vi "Kikusui PLZ-Configure Operation Value.vi"(8 "error in":errorcluster, 9 "Values (0)":dbl format="%#.3g", 10 "Value Type (0:Current)":u16(ring) items=["Current", "Voltage", "Power", "Conductance"], 11 "Kikusui PLZ Setting In":T1={"VISA Resource Name"="", "Baud Rate"=19200, "Stop Bits"=20, "Wait For Read(ms)"=0} {"Stop Bits" items=["1.0"=10, "2.0"=20]; "Baud Rate" items=["2400"=2400, "4800"=4800, "9600"=9600, "19200"=19200]}) -> (0 "error out":errorcluster, 3 "Kikusui PLZ Setting Out":T1={"VISA Resource Name"="", "Baud Rate"=19200, "Stop Bits"=20, "Wait For Read(ms)"=0} {"Stop Bits" items=["1.0"=10, "2.0"=20]; "Baud Rate" items=["2400"=2400, "4800"=4800, "9600"=9600, "19200"=19200]})   [LabVIEW 2018]
doc: "Configures the current, voltage, power or conductance depending the instrument operation mode.\n\n<b>Note:</b>\nIn these modes, only the following values are allowed.\n1) CC -Current\n2) CV -Voltage\n3) CP -Power\n4) CR- Conductance\n5) CC+CV -Current & Voltage\n6) CR+CV -Conductance & Voltage"
uses:
  Data Def/Kikusui PLZ-Setting.ctl
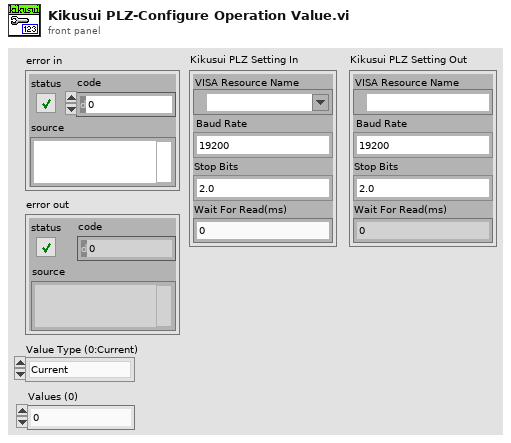
[diagram p1: front panel]
types:
  T1 = typedef "Kikusui PLZ-Setting.ctl" = cluster{"VISA Resource Name":refnum<visa-resource-name>, "Baud Rate":u32, "Stop Bits":u16, "Wait For Read(ms)":u32}
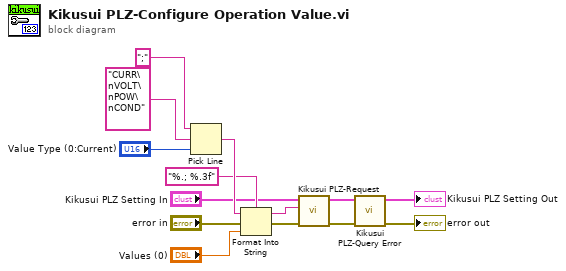
[diagram p0: block diagram]
diagram:
  n1 = Pick Line(string ("")=";", multi-line string="CURR\nVOLT\nPOW\nCOND", line index="Value Type (0:Current)") -> (output string=w12:string)
  n2 = Format Into String(format string="%.; %.3f", initial string=w12, error in="error in", "Values (0)") -> (resulting string=w6:string, error out=w7:errorcluster)
  n3 = call "Kikusui PLZ-Request.vi"("error in"=w7, "Command"=w6, "Kikusui PLZ Setting In"="Kikusui PLZ Setting In") -> ("error out"=w5:errorcluster, "Kikusui PLZ Setting Out"=w4:T1)  [unwired: 6 in, 1 out]
  n4 = call "Kikusui PLZ-Query Error.vi"("error in"=w5, "Kikusui PLZ Setting In"=w4) -> ("error out"=→"error out":errorcluster, "Kikusui PLZ Setting Out"=→"Kikusui PLZ Setting Out":T1)  [unwired: 8 in]
